vi "Read Termination Message.vi"(0 "message queue in":T3, 1 "ignore error on termination message (F)":bool, 5 "timeout (1 ms)":i32=1, 9 "termination list ([Exit])":string[](array[string])=["Exit"]) -> (3 "termination message":bool, 4 "message queue out":T3, 12 "message":T1)   [LabVIEW 2015, in "Car Wash.lvlib" / "AMC.lvlib"]
uses:
  AMC.lvlib
  Tools/Keyed Array/KeyedArray.ctl
  Tools/Keyed Array/Tools_KeyedArray.lvlib
  Message.ctl
  Message Queue.ctl
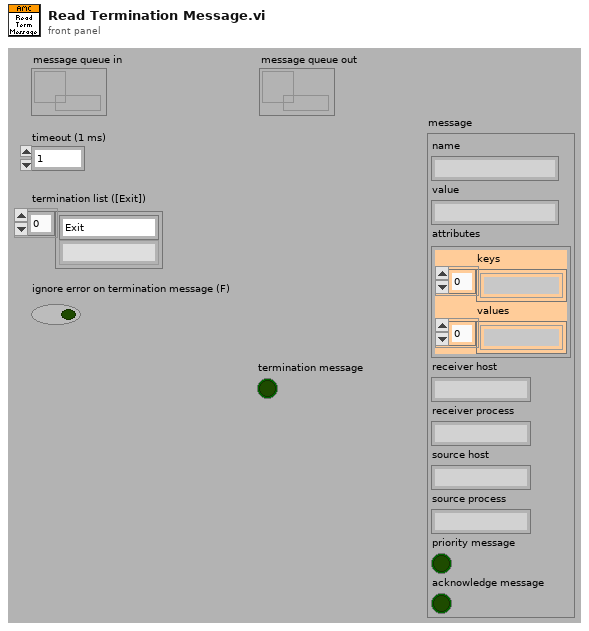
[diagram p1: front panel]
types:
  T1 = typedef "Car Wash.lvlib/AMC.lvlib/Message.ctl" = cluster{"name":string, "value":string, "attributes":T2, "receiver host":string, "receiver process":string, "source host":string, "source process":string, "priority message":bool, "acknowledge message":bool}
  T2 = typedef "Car Wash.lvlib/Tools_KeyedArray.lvlib/KeyedArray.ctl" = cluster{"keys":string[], "values":string[]}
  T3 = typedef "Car Wash.lvlib/AMC.lvlib/Message Queue.ctl" = refnum<queue>
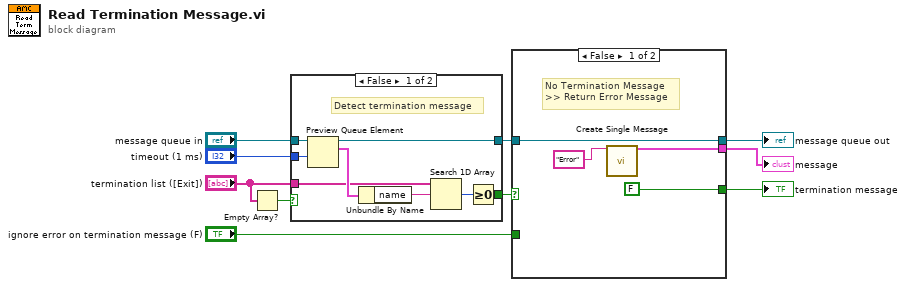
[diagram p0: block diagram]
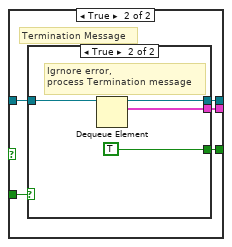
[diagram p3: hidden frame]
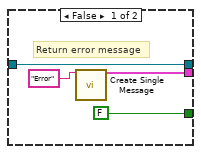
[diagram p4: hidden frame]
diagram:
  n1 = Empty Array?(array="termination list ([Exit])") -> (empty?=w1:bool)
  n2 = case shown="False" w1 {
    tunnel: "message queue in" -> [w18 w19]
    tunnel: "timeout (1 ms)" -> [w17 _]
    tunnel: [w13 _] -> w7
    tunnel: [w12 w19] -> w6
    tunnel: "termination list ([Exit])" -> [w11 _]
    frame False {
      # "Detect termination message"
      n3 = Preview Queue Element(queue=w18, timeout in ms (-1)=w17) -> (queue out=w12:T3, element=w16:T1)  [unwired: 1 in, 2 out]
      n4 = Unbundle By Name(w16) -> ("name"=w14:string)
      n5 = Search 1D Array(1D array=w11, element=w14) -> (index of element=w15:i32)  [unwired: 1 out]
      n6 = Greater Or Equal To 0?(x=w15) -> (x >= 0?=w13:bool)
    }
    frame True {
    }
  }
  n7 = case shown="False" w7 {
    tunnel: [FALSE w26] -> w3
    tunnel: [w22 w25] -> w5
    tunnel: w6 -> [w22 w28]
    tunnel: "ignore error on termination message (F)" -> [_ w27]
    tunnel: [w20 w24] -> w4
    frame False {
      # "No Termination Message\n>> Return Error Message"
      n8 = call "Create Single Message.vi"("name"="Error") -> ("message"=w20:T1)  [unwired: 13 in, 1 out]
    }
    frame True {
      # "Termination Message"
      n9 = case shown="True" w27 {
        tunnel: w28 -> [w31 w36]
        tunnel: [FALSE TRUE] -> w26
        tunnel: [w31 w33] -> w25
        tunnel: [w30 w34] -> w24
        frame False {
          # "Return error message"
          n10 = call "Create Single Message.vi"("name"="Error") -> ("message"=w30:T1)  [unwired: 13 in, 1 out]
        }
        frame True {
          # "Igrnore error,\nprocess Termination message"
          n11 = Dequeue Element(queue=w36) -> (queue out=w33:T3, element=w34:T1)  [unwired: 2 in, 2 out]
        }
      }
    }
  }
  "message queue out" <- w5
  "message" <- w4
  "termination message" <- w3
